vi "NI PXI-4110 Programmable Power Supply Main Page.vi"(8 "error in (no error)":errorcluster, 11 "Node Ptr":T2 format="%.0x") -> (0 "error out":errorcluster)   [LabVIEW 2018, in "NI PXI-4110 Programmable Power Supply Custom Device.lvlib"]
uses:
  NI PXI-4110 Programmable Power Supply Custom Device.lvlib
  <vilib>/NI Veristand/Custom Device API/Custom Device Item Ref.ctl
  Power_Supply_In_Use.ctl
  4110_Global.vi
  <vilib>/NI Veristand/Custom Device API/Get Item Property (String).vi
  <vilib>/NI Veristand/Custom Device API/Get Item Property (U16).vi
  <vilib>/NI Veristand/Custom Device API/Set Item Property (Boolean).vi
  <vilib>/NI Veristand/Custom Device API/Get Item Property (Boolean).vi
  <vilib>/NI Veristand/Custom Device API/Set Item Property (String).vi
  <vilib>/NI Veristand/Custom Device API/Set Item Property (U16).vi
  <vilib>/NI VeriStand/Custom Device API/Custom Device API.lvlib
panel:
  in  "Power Supply In Use":T1
  in  "Power Source":bool
  in  "Power Supply NI-MAX Device Name":string
  in  "Add Current Chans":bool
  in  "Header":cluster{"Section Name":string}={"Section Name"="PXI-4110  Settings"}
  in  "Description":string
  in  "Custom Device Name":string
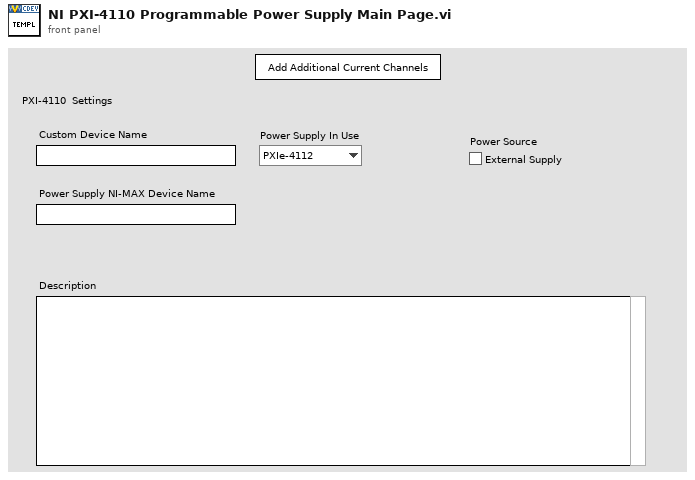
[diagram p1: front panel]
types:
  T1 = typedef "NI PXI-4110 Programmable Power Supply Custom Device.lvlib/Power_Supply_In_Use.ctl" = enum16{"PXIe-4112", "PXI-4110"}
  T2 = typedef "Custom Device API.lvlib/Custom Device Item Ref.ctl" = u64
  T3 = enum8{"Enabled", "Disabled", "Disabled and Grayed Out"}
  T4 = typedef "Custom Device API.lvlib/Custom Device Item Info.ctl" = cluster{"Name":string, "Is Channel":bool, "GUID":string, "Is Waveform":bool}
  T5 = typedef "Custom Device API.lvlib/Custom Device Commands.ctl" = enum16{"Default", "Item renamed", "Shutdown", "Dynamic button pressed"}
  T6 = typedef "niDCPower Sense.ctl" = i32
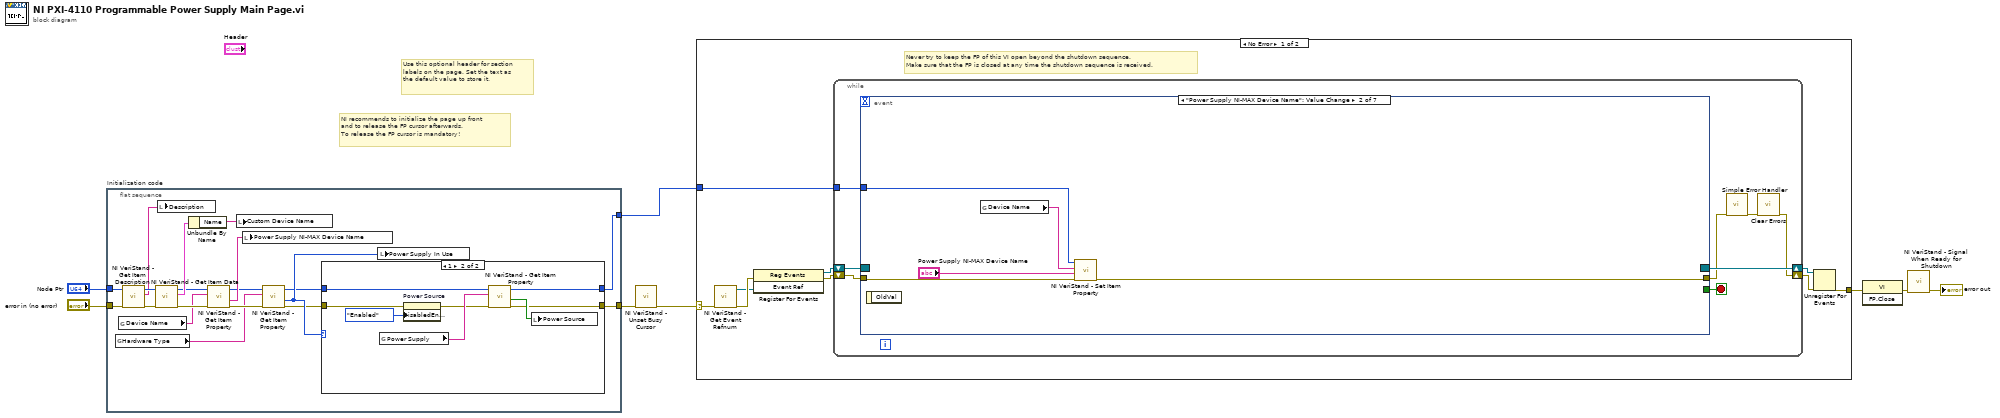
[diagram p0: block diagram]
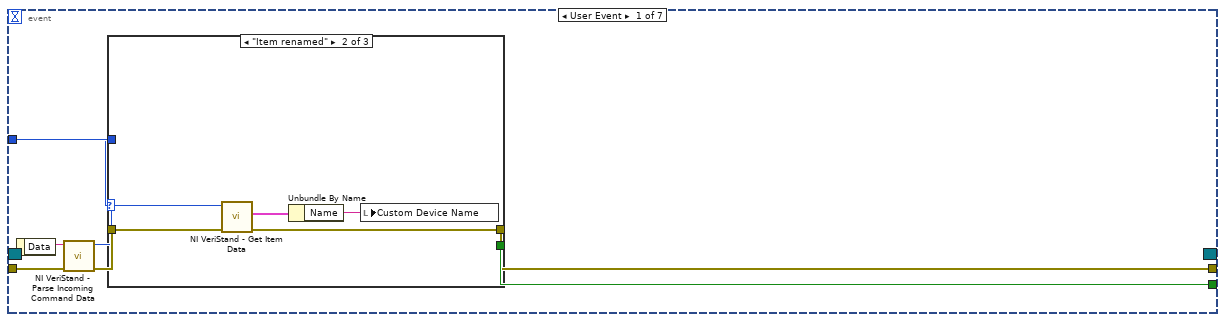
[diagram p2: hidden frame]
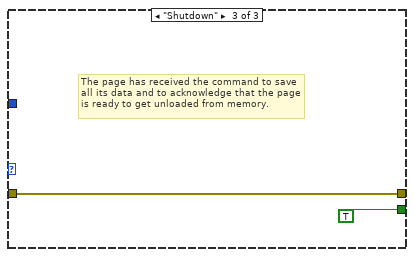
[diagram p4: hidden frame]
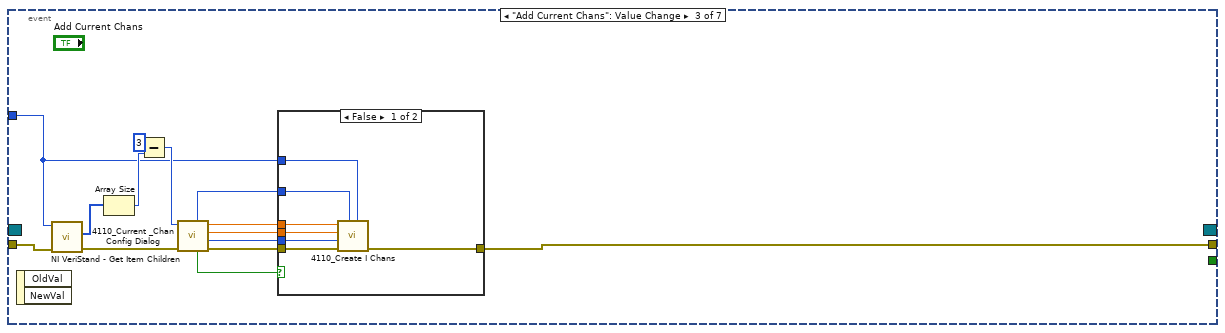
[diagram p5: hidden frame]
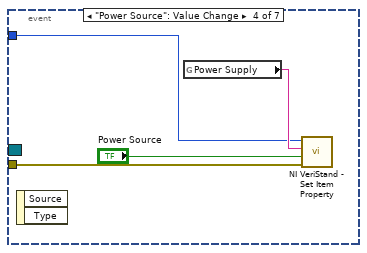
[diagram p7: hidden frame]
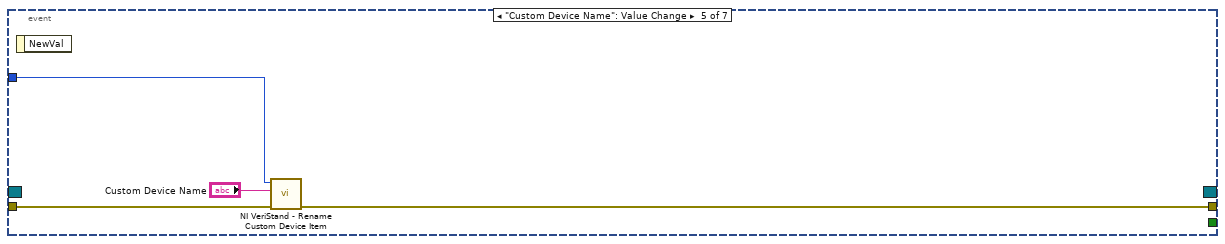
[diagram p8: hidden frame]
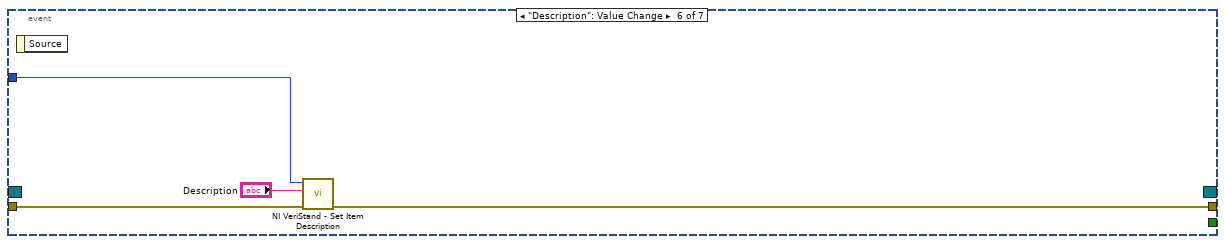
[diagram p9: hidden frame]
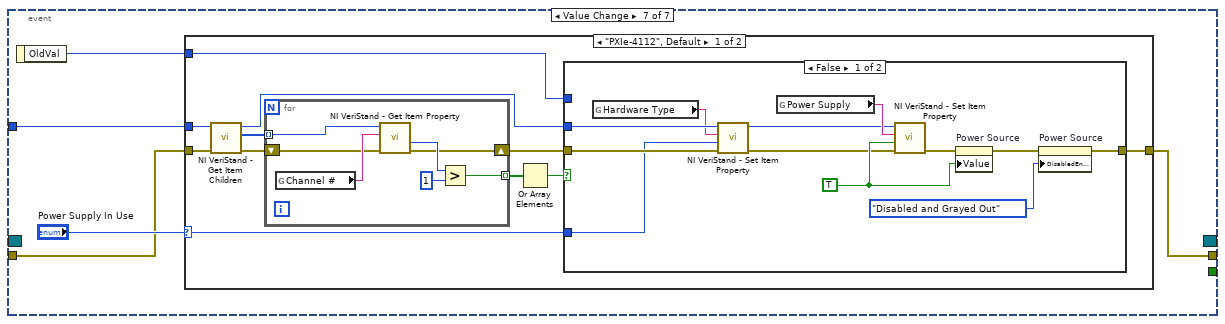
[diagram p10: hidden frame]
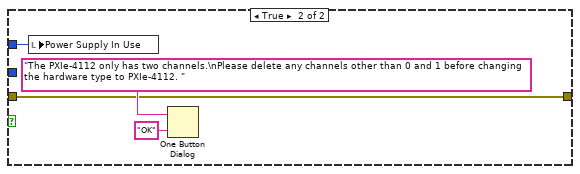
[diagram p11: hidden frame]
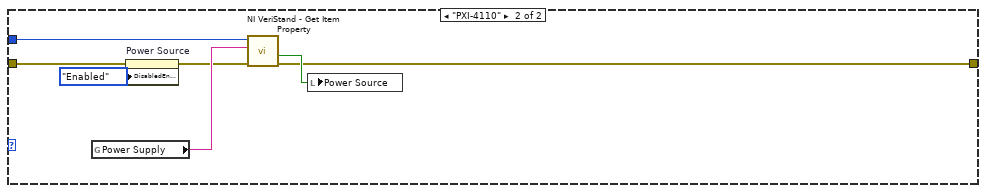
[diagram p12: hidden frame]
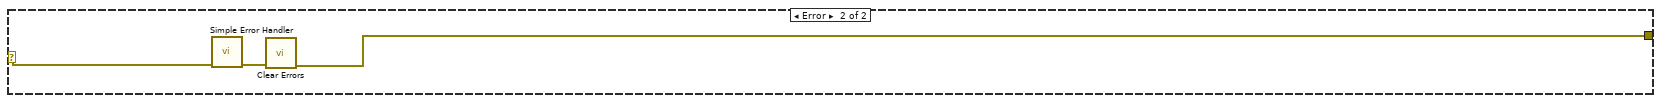
[diagram p13: hidden frame]
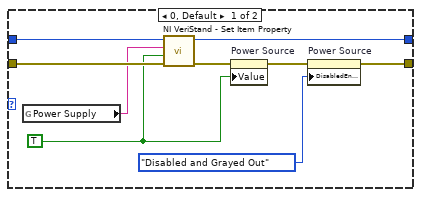
[diagram p14: hidden frame]
diagram:
  # "Use this optional header for section labels on the page. Set the text as the default value to store it."
  # "NI recommends to initialize the page up front\nand to release the FP cursor afterwards.\nTo release the FP cursor is mandatory!"
  n1 = flat-sequence "Initialization code" {
    tunnel: "error in (no error)" -> [w21]
    tunnel: "Node Ptr" -> [w22]
    tunnel: [w9] -> w4
    tunnel: [w11] -> w1
    frame #0 {
      n2 = global read "4110_Global.vi" "Hardware Type"() -> (w14:string)
      n3 = global read "4110_Global.vi" "Device Name"() -> (w18:string)
      n4 = call <vilib>:"NI VeriStand - Get Item Description.vi"("error in (no error)"=w21, "Item Ref in"=w22) -> ("error out"=w25:errorcluster, "Description"=w26:string, "Item Ref out"=w27:T2)  [unwired: 7 out]
      n5 = call <vilib>:"NI VeriStand - Get Item Data.vi"("error in (no error)"=w25, "Item Ref in"=w27) -> ("error out"=w20:errorcluster, "Item Info"=w24:T4, "Item Ref out"=w19:T2)  [unwired: 7 out]
      n6 = local write "Description"(w26) -> ()
      n7 = Unbundle By Name(w24) -> ("Name"=w23:string)
      n8 = call-poly <vilib>:"NI VeriStand - Get Item Property.vi"("error in (no error)"=w20, "Property Name"=w18, "Item Ref in"=w19) -> ("error out"=w15:errorcluster, "Value"=w17:string, "Item Ref out"=w16:T2)  [unwired: 5 in, 1 out]
      n9 = local write "Custom Device Name"(w23) -> ()
      n10 = local write "Power Supply NI-MAX Device Name"(w17) -> ()
      n11 = call-poly <vilib>:"NI VeriStand - Get Item Property.vi"("error in (no error)"=w15, "Property Name"=w14, "Item Ref in"=w16) -> ("error out"=w10:errorcluster, "Value"=w13:u16, "Item Ref out"=w12:T2)  [unwired: 5 in, 1 out]
      n12 = case shown="1" w13 {
        tunnel: [w28 w44] -> w11
        tunnel: w12 -> [w33 w41]
        tunnel: w10 -> [w32 w39]
        tunnel: [w36 w40] -> w9
        frame 0, Default {
          w30 = TRUE ("Power Source")
          n13 = global read "4110_Global.vi" "Power Supply"() -> (w31:string)
          n14 = call-poly <vilib>:"NI VeriStand - Set Item Property.vi"("error in (no error)"=w32, "Value"=w30, "Property Name"=w31, "Item Ref in"=w33) -> ("error out"=w29:errorcluster, "Item Ref out"=w28:T2)  [unwired: 5 in, 1 out]
          n15 = property on="Power Source" class="Bool (strict)"(error in=w29, "Value"=w30) -> (error out=w34:errorcluster)  [unwired: 1 in, 1 out]
          n16 = property on="Power Source" class="Bool (strict)"(error in=w34, "DisabledEnum"=T3."Disabled and Grayed Out" ("Disabled")) -> (error out=w36:errorcluster)  [unwired: 1 in, 1 out]
        }
        frame 1 {
          n17 = global read "4110_Global.vi" "Power Supply"() -> (w43:string)
          n18 = property on="Power Source" class="Bool (strict)"(error in=w39, "DisabledEnum"=T3."Enabled" ("Disabled")) -> (error out=w38:errorcluster)  [unwired: 1 in, 1 out]
          n19 = call-poly <vilib>:"NI VeriStand - Get Item Property.vi"("error in (no error)"=w38, "Property Name"=w43, "Item Ref in"=w41) -> ("error out"=w40:errorcluster, "Value"=w42:bool, "Item Ref out"=w44:T2)  [unwired: 5 in, 1 out]
          n20 = local write "Power Source"(w42) -> ()
        }
      }
      n21 = local write "Power Supply In Use"(w13) -> ()
    }
  }
  n22 = call <vilib>:"NI VeriStand - Unset Busy Cursor.vi"("error in (no error)"=w4) -> ("error out"=w3:errorcluster)  [unwired: 10 out]
  n23 = case shown="No Error" w3 {
    selector: w3 -> [w45 w164]
    tunnel: [w50 w162] -> w8
    tunnel: w1 -> [w46 _]
    frame No Error {
      # "Never try to keep the FP of this VI open beyond the shutdown sequence.\nMake sure that the FP is closed at any time the shutdown sequence is received."
      n24 = call <vilib>:"NI VeriStand - Get Event Refnum.vi"("error in (no error)"=w45) -> ("error out"=w53:errorcluster, "Event Ref"=w49:refnum<user-event>)  [unwired: 9 out]
      n25 = register-events(error in=w53, w49) -> (reference out=w47:refnum<event-registration>, error out=w48:errorcluster)  [unwired: 1 in]
      n26 = while {
        tunnel: w46 -> [w57]
        shift-right: [w54] -> w51
        shift-left: w48 -> [w60]
        shift-right: [w61] -> w52
        shift-left: w47 -> [w59]
        stop <- w58 stop-if-true
        n27 = event shown="[1] \"Power Supply NI-MAX Device Name\": Value Change" {
          selector: w59 -> [_ _ _ _ _ _ _]
          dyn-events: [_ _ _ _ _ _ _] -> w61
          timeout: _ -> [_ _ _ _ _ _ _]
          tunnel: w60 -> [w68 w81 w95 w104 w111 w114 w118]
          tunnel: [w64 _ _ _ _ _ _] -> w58
          tunnel: [w63 w77 w83 _ w110 w113 w120] -> w56
          tunnel: w57 -> [w62 w80 w89 w106 w109 w115 w117]
          event User Event {
            n28 = event-data() -> ("Data"=w67:string)  [unwired: 1 out]
            n29 = call <vilib>:"NI VeriStand - Parse Incoming Command Data.vi"("error in (no error)"=w68, "Incoming data"=w67) -> ("error out"=w66:errorcluster, "Action"=w65:T5)  [unwired: 8 out]
            n30 = case shown="\"Item renamed\"" w65 {
              tunnel: w66 -> [w69 w74 w75]
              tunnel: [_ _ TRUE] -> w64
              tunnel: [w69 w71 w75] -> w63
              tunnel: w62 -> [_ w73 _]
              frame "Default", Default {
              }
              frame "Item renamed" {
                n31 = call <vilib>:"NI VeriStand - Get Item Data.vi"("error in (no error)"=w74, "Item Ref in"=w73) -> ("error out"=w71:errorcluster, "Item Info"=w72:T4)  [unwired: 8 out]
                n32 = Unbundle By Name(w72) -> ("Name"=w70:string)
                n33 = local write "Custom Device Name"(w70) -> ()
              }
              frame "Shutdown" {
                # "The page has received the command to save all its data and to acknowledge that the page is ready to get unloaded from memory."
              }
            }
          }
          event "Power Supply NI-MAX Device Name": Value Change {
            n34 = event-data() -> ()  [unwired: 2 out]
            n35 = global read "4110_Global.vi" "Device Name"() -> (w79:string)
            n36 = call-poly <vilib>:"NI VeriStand - Set Item Property.vi"("error in (no error)"=w81, "Value"="Power Supply NI-MAX Device Name", "Property Name"=w79, "Item Ref in"=w80) -> ("error out"=w77:errorcluster)  [unwired: 5 in, 2 out]
          }
          event "Add Current Chans": Value Change {
            n37 = event-data() -> ()  [unwired: 3 out]
            n38 = call <vilib>:"NI VeriStand - Get Item Children.vi"("error in (no error)"=w95, "Item Ref in"=w89) -> ("error out"=w94:errorcluster, "Child Refs"=w82:T2[])  [unwired: 6 in, 2 out]
            n39 = Array Size(array=w82) -> (size(s)=w92:i32)
            n40 = Subtract(x=3, y=w92) -> (x-y=w91:i32)
            n41 = call "4110_Current _Chan Config Dialog.vi"("error in (no error)"=w94, "Data Entry Limits:Maximum"=w91) -> ("error out"=w84:errorcluster, "sense (out)"=w85:T6, "Voltage Limit (out)"=w86:dbl, "Initial Current Value (out)"=w87:dbl, "Cancel (out)"=w90:bool, "Number of Current Channels to Add? (out)"=w88:i16)  [unwired: 4 in]
            n42 = case shown="False" w90 {
              tunnel: w89 -> [w102 _]
              tunnel: w88 -> [w101 _]
              tunnel: w87 -> [w100 _]
              tunnel: w86 -> [w99 _]
              tunnel: w85 -> [w98 _]
              tunnel: w84 -> [w97 w103]
              tunnel: [w96 w103] -> w83
              frame False {
                n43 = call "4110_Create I Chans.vi"("Device Ref in"=w102, "# of I Channels to Add?"=w101, "error in"=w97, "sense"=w98, "Voltage Limit"=w99, "Init Value"=w100) -> ("error out"=w96:errorcluster)  [unwired: 5 in]
              }
              frame True {
                # "Canceled"
              }
            }
          }
          event "Power Source": Value Change {
            n44 = event-data() -> ()  [unwired: 3 out]
            n45 = global read "4110_Global.vi" "Power Supply"() -> (w107:string)
            n46 = call-poly <vilib>:"NI VeriStand - Set Item Property.vi"("error in (no error)"=w104, "Value"="Power Source", "Property Name"=w107, "Item Ref in"=w106) -> ()  [unwired: 5 in, 3 out]
          }
          event "Custom Device Name": Value Change {
            n47 = event-data() -> ()  [unwired: 2 out]
            n48 = call <vilib>:"NI VeriStand - Rename Custom Device Item.vi"("error in (no error)"=w111, "New Name"="Custom Device Name", "Item Ref in"=w109) -> ("error out"=w110:errorcluster)  [unwired: 1 in, 7 out]
          }
          event "Description": Value Change {
            n49 = event-data() -> ()  [unwired: 2 out]
            n50 = call <vilib>:"NI VeriStand - Set Item Description.vi"("error in (no error)"=w114, "Description"="Description", "Item Ref in"=w115) -> ("error out"=w113:errorcluster)  [unwired: 8 out]
          }
          event Value Change {
            n51 = event-data() -> ("OldVal"=w116:T1)  [unwired: 1 out]
            n52 = case shown="\"PXIe-4112\", Default" "Power Supply In Use" {
              selector: "Power Supply In Use" -> [w122 _]
              tunnel: w117 -> [w129 w159]
              tunnel: w118 -> [w128 w157]
              tunnel: [w121 w158] -> w120
              tunnel: w116 -> [w125 _]
              frame "PXIe-4112", Default {
                n53 = call <vilib>:"NI VeriStand - Get Item Children.vi"("error in (no error)"=w128, "Item Ref in"=w129) -> ("error out"=w130:errorcluster, "Child Refs"=w131:T2[], "Item Ref out"=w124:T2)  [unwired: 6 in, 1 out]
                n54 = for {
                  tunnel: w131 -> [w154] mode=indexing
                  tunnel: [w149] -> w127 mode=indexing
                  shift-right: [w148] -> w123
                  shift-left: w130 -> [w152]
                  n55 = global read "4110_Global.vi" "Channel #"() -> (w153:string)
                  n56 = call-poly <vilib>:"NI VeriStand - Get Item Property.vi"("error in (no error)"=w152, "Property Name"=w153, "Item Ref in"=w154) -> ("error out"=w148:errorcluster, "Value"=w151:u16)  [unwired: 5 in, 2 out]
                  n57 = Greater?(x=w151, y=u16 1) -> (0:w149:bool)
                }
                n58 = Or Array Elements(Boolean array=w127) -> (logical OR=w126:bool)
                n59 = case shown="False" w126 {
                  tunnel: w125 -> [_ w145]
                  tunnel: w124 -> [w138 _]
                  tunnel: w123 -> [w137 w144]
                  tunnel: w122 -> [w135 _]
                  tunnel: [w132 w144] -> w121
                  frame False {
                    w140 = TRUE ("Power Source")
                    n60 = global read "4110_Global.vi" "Hardware Type"() -> (w136:string)
                    n61 = call-poly <vilib>:"NI VeriStand - Set Item Property.vi"("error in (no error)"=w137, "Value"=w135, "Property Name"=w136, "Item Ref in"=w138) -> ("error out"=w133:errorcluster, "Item Ref out"=w134:T2)  [unwired: 5 in, 1 out]
                    n62 = global read "4110_Global.vi" "Power Supply"() -> (w142:string)
                    n63 = call-poly <vilib>:"NI VeriStand - Set Item Property.vi"("error in (no error)"=w133, "Value"=w140, "Property Name"=w142, "Item Ref in"=w134) -> ("error out"=w141:errorcluster)  [unwired: 5 in, 2 out]
                    n64 = property on="Power Source" class="Bool (strict)"(error in=w141, "Value"=w140) -> (error out=w143:errorcluster)  [unwired: 1 in, 1 out]
                    n65 = property on="Power Source" class="Bool (strict)"(error in=w143, "DisabledEnum"=T3."Disabled and Grayed Out" ("Disabled")) -> (error out=w132:errorcluster)  [unwired: 1 in, 1 out]
                  }
                  frame True {
                    n66 = local write "Power Supply In Use"(w145) -> ()
                    n67 = One Button Dialog(message="The PXIe-4112 only has two channels.\nPlease delete any channels other than 0 and 1 before changing the hardware type to PXIe-4112. ", button name ("OK")="OK") -> ()  [unwired: 1 out]
                  }
                }
              }
              frame "PXI-4110" {
                n68 = global read "4110_Global.vi" "Power Supply"() -> (w161:string)
                n69 = property on="Power Source" class="Bool (strict)"(error in=w157, "DisabledEnum"=T3."Enabled" ("Disabled")) -> (error out=w156:errorcluster)  [unwired: 1 in, 1 out]
                n70 = call-poly <vilib>:"NI VeriStand - Get Item Property.vi"("error in (no error)"=w156, "Property Name"=w161, "Item Ref in"=w159) -> ("error out"=w158:errorcluster, "Value"=w160:bool)  [unwired: 5 in, 2 out]
                n71 = local write "Power Source"(w160) -> ()
              }
            }
          }
        }
        n72 = call <vilib>:"Simple Error Handler.vi"("error in (no error)"=w56) -> ("error out"=w55:errorcluster)  [unwired: 1 in, 7 out]
        n73 = call <vilib>:"Clear Errors.vi"("error in (no error)"=w55) -> ("error out"=w54:errorcluster)  [unwired: 1 in, 5 out]
      }
      n74 = Unregister For Events(event registration refnum=w52, error in=w51) -> (error out=w50:errorcluster)
    }
    frame Error {
      n75 = call <vilib>:"Simple Error Handler.vi"("error in (no error)"=w164) -> ("error out"=w163:errorcluster)  [unwired: 1 in, 7 out]
      n76 = call <vilib>:"Clear Errors.vi"("error in (no error)"=w163) -> ("error out"=w162:errorcluster)  [unwired: 1 in, 5 out]
    }
  }
  n77 = invoke class="VI" method="FP.Close"(error in=w8) -> (error out=w7:errorcluster)  [unwired: 2 in, 2 out]
  n78 = call <vilib>:"NI VeriStand - Signal When Ready for Shutdown.vi"("error in (no error)"=w7) -> ("error out"=→"error out":errorcluster)  [unwired: 10 out]
